vi "Read Data.vi"(8 "error in (no error)":errorcluster, 11 "TDMS in":refnum<class "TDMS.lvclass">) -> (0 "error out":errorcluster, 2 "data":waveform(dbl)[](array[waveform]), 3 "TDMS out":refnum<class "TDMS.lvclass">)   [LabVIEW 2020, in "TDMS.lvclass"]
uses:
  TDMS.lvclass
  TDMS.lvclass/TDMS.ctl
  Abstrut Data/Abstruct Data Type.lvclass/Abstruct Data Type.ctl
  Abstrut Data/Accessors/Read Index.vi
  Abstrut Data/Accessors/Read Range.vi
  Abstrut Data/Accessors/Read Selected Channels.vi
  Abstrut Data/Accessors/Read Table Names.vi
  Abstrut Data/Accessors/Read Selected Table.vi
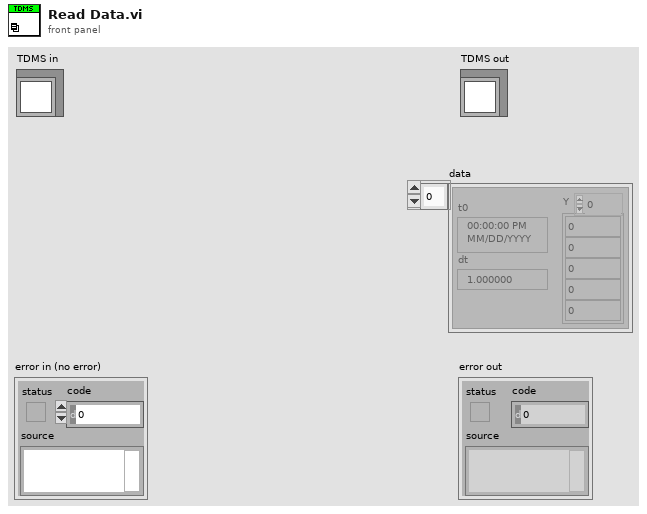
[diagram p1: front panel]
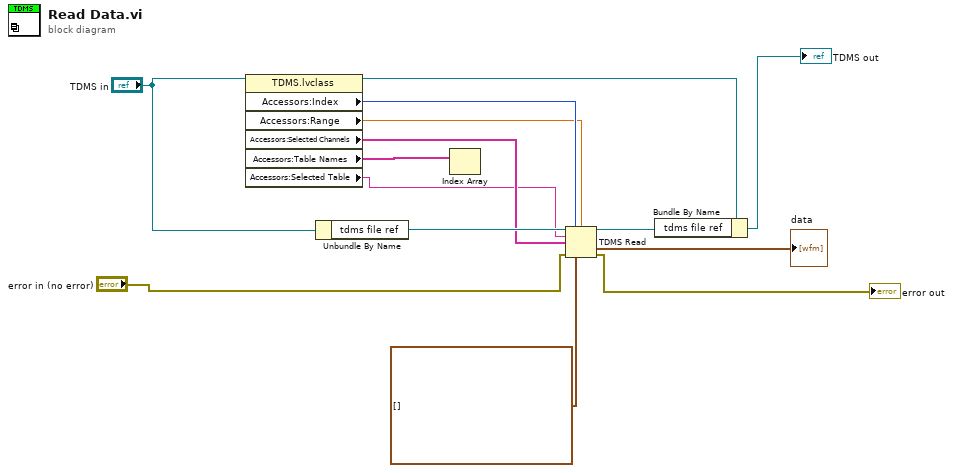
[diagram p0: block diagram]
diagram:
  n1 = property on="Property Node" class="TDMS.lvclass"(reference="TDMS in") -> (reference out=w7:refnum<class "TDMS.lvclass">, "Accessors:Index"=w12:u64, "Accessors:Range"=w11:dbl, "Accessors:Selected Channels"=w10:string[], "Accessors:Table Names"=w2:string[], "Accessors:Selected Table"=w1:string)  [unwired: 1 in, 1 out]
  n2 = Unbundle By Name("TDMS in") -> ("tdms file ref"=w14:refnum<k34>)
  n3 = Index Array(array=w2) -> ()  [unwired: 1 in, 1 out]
  n4 = TDMS Read(0:w14, 1:w12, 2:w11, 5:w1, 7:w10, 11:"error in (no error)", 12:waveform(dbl)[] [] ("data type")) -> (4:w6:refnum<k34>, 10:→"data":waveform(dbl)[], 15:→"error out":errorcluster)  [unwired: 1 in, 3 out]
  n5 = Bundle By Name(cluster=w7, "tdms file ref"=w6) -> (→"TDMS out":refnum<class "TDMS.lvclass">)
